vi "GetGrowableFunctions.vi"(6 "error in":errorcluster, 9 "Diagram in":refnum<class "Diagram.lvclass">) -> (0 "error out":errorcluster, 3 "Diagram out":refnum<class "Diagram.lvclass">, 4 "growable functions":i32[](array[numeric]))   [LabVIEW 2014, in "Raspberry Pi Compatible Compiler for LabVIEW.lvlib" / "Diagram.lvclass"]
uses:
  Diagram.lvclass
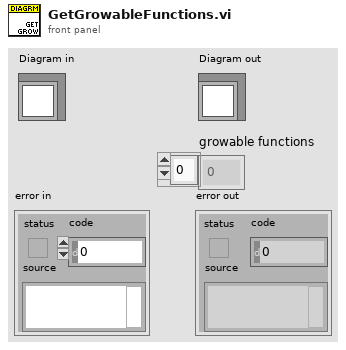
[diagram p1: front panel]
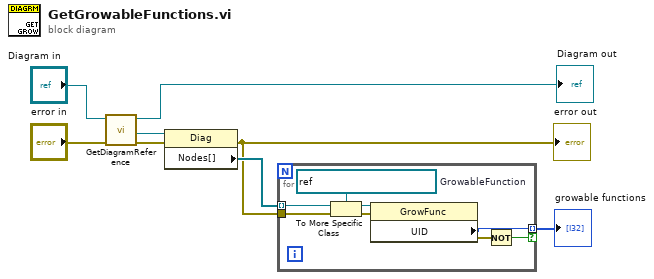
[diagram p0: block diagram]
diagram:
  n1 = call "GetDiagramReference.vi"("error in"="error in", "Diagram in"="Diagram in") -> ("error out"=w5:errorcluster, "reference out"=w4:refnum<vi>, "Diagram out"=→"Diagram out":refnum<class "Diagram.lvclass">)  [unwired: 5 in]
  n2 = property class="Diag"(reference=w4, error in=w5) -> (error out=w2:errorcluster, "Nodes[]"=w3:refnum<vi>[])  [unwired: 1 out]
  "error out" <- w2
  n3 = for {
    tunnel: w3 -> [w9] mode=indexing
    tunnel: w2 -> [w16]
    tunnel: [w12] -> w1 mode=indexing if=w10
    w15 = refnum<vi> refnum  # GrowableFunction
    n4 = To More Specific Class(target class=w15, reference=w9, error in=w16) -> (specific class reference=w14:refnum<vi>, error out=w13:errorcluster)
    n5 = property class="GrowFunc"(reference=w14, error in=w13) -> (error out=w11:errorcluster, "UID"=w12:i32)  [unwired: 1 out]
    n6 = Not(x=w11) -> (.not. x?=w10:bool)
  }
  "growable functions" <- w1
